vi "Write Horizontal Scrollbar Visibility.vi"(5 "Horizontal Scrollbar Visibility":T1(ring), 9 "Pane in":refnum<class "Pane.lvclass">) -> (3 "Pane out":refnum<class "Pane.lvclass">)   [LabVIEW 2014, in "Raspberry Pi Compatible Compiler for LabVIEW.lvlib" / "Pane.lvclass"]
uses:
  Pane.lvclass
  Pane.lvclass/Pane.ctl
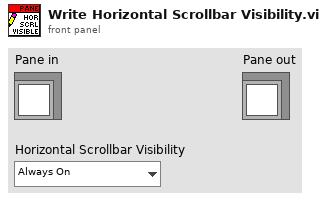
[diagram p1: front panel]
types:
  T1 = enum16{"Always On", "Always Off", "Off While Running"}
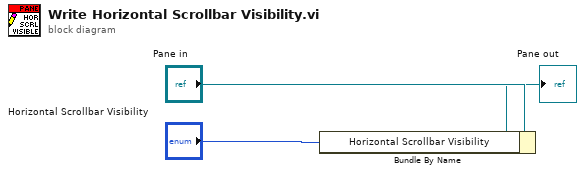
[diagram p0: block diagram]
diagram:
  n1 = Bundle By Name(cluster="Pane in", "Horizontal Scrollbar Visibility"="Horizontal Scrollbar Visibility") -> (→"Pane out":refnum<class "Pane.lvclass">)
